vi "FGV_RichText.vi"(11 ".NET Refnum in":refnum<k24>) -> ()   [LabVIEW 2017]
uses:
  System.Windows.Forms
panel:
  out "error out":errorcluster
  in  "error in (no error)":errorcluster
  in  "FV":T1(ring)
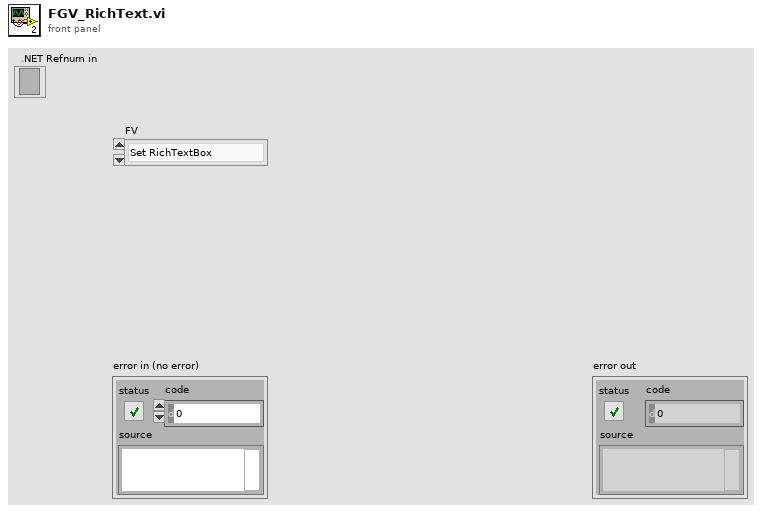
[diagram p1: front panel]
types:
  T1 = enum16{"Set RichTextBox", "LoadRTFFile", "Undo", "Redo", "Copy", "Cut", "Past", "Clear", "Find", "Save", "Initialize"}
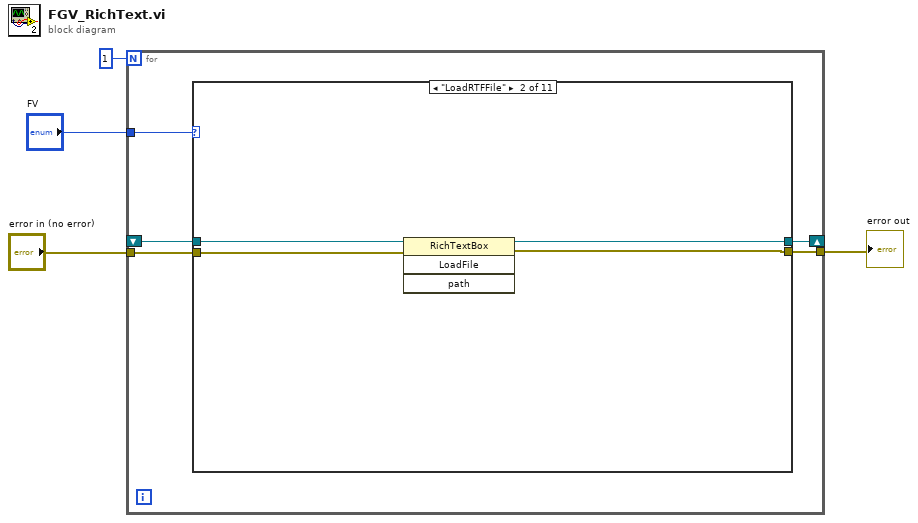
[diagram p0: block diagram]
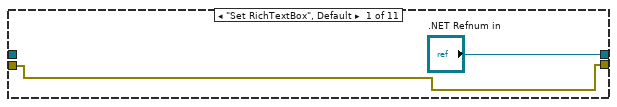
[diagram p2: hidden frame]
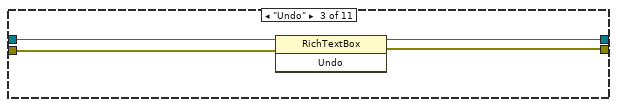
[diagram p3: hidden frame]
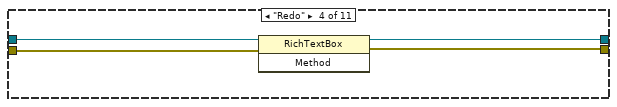
[diagram p4: hidden frame]
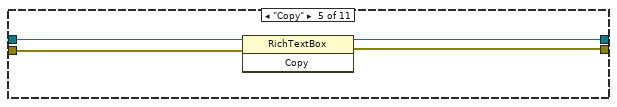
[diagram p5: hidden frame]
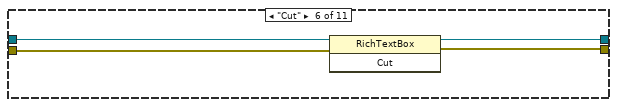
[diagram p6: hidden frame]
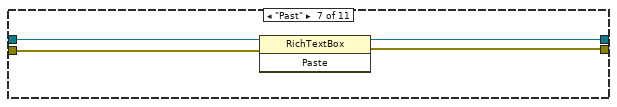
[diagram p7: hidden frame]
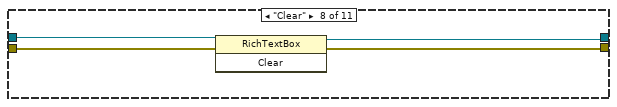
[diagram p8: hidden frame]
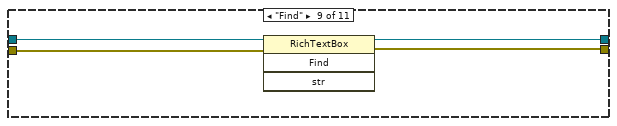
[diagram p9: hidden frame]
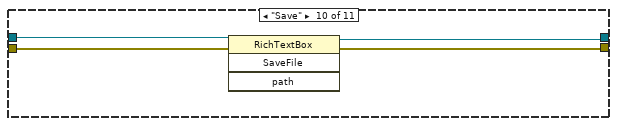
[diagram p10: hidden frame]
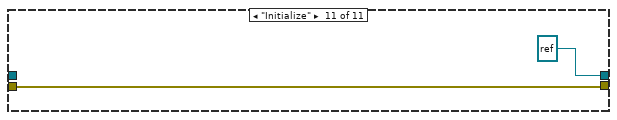
[diagram p11: hidden frame]
diagram:
  n1 = for {
    N: 1 -> [_]
    tunnel: "FV" -> [w9]
    shift-right: [w8] -> _
    shift-left: _ -> [w7]
    tunnel: [w6] -> w2
    tunnel: "error in (no error)" -> [w5]
    n2 = case shown="\"LoadRTFFile\"" w9 {
      tunnel: [".NET Refnum in" w12 w18 w21 w25 w29 w33 w37 w41 w45 refnum<k24> refnum (".NET Refnum in")] -> w8
      tunnel: w7 -> [_ w15 w19 w23 w27 w31 w35 w39 w43 w47 _]
      tunnel: [w10 w14 w17 w20 w24 w28 w32 w36 w40 w44 w49] -> w6
      tunnel: w5 -> [w10 w13 w16 w22 w26 w30 w34 w38 w42 w46 w49]
      frame "Set RichTextBox", Default {
      }
      frame "LoadRTFFile" {
        n3 = invoke class="RichTextBox" method="LoadFile"(reference=w15, error in=w13) -> (reference out=w12:refnum<k24>, error out=w14:errorcluster)  [unwired: 2 in, 2 out]
      }
      frame "Undo" {
        n4 = invoke class="RichTextBox" method="Undo"(reference=w19, error in=w16) -> (reference out=w18:refnum<k24>, error out=w17:errorcluster)  [unwired: 1 in, 1 out]
      }
      frame "Redo" {
        n5 = invoke class="RichTextBox" method=#-1(reference=w23, error in=w22) -> (reference out=w21:refnum<k24>, error out=w20:errorcluster)  [unwired: 1 in, 1 out]
      }
      frame "Copy" {
        n6 = invoke class="RichTextBox" method="Copy"(reference=w27, error in=w26) -> (reference out=w25:refnum<k24>, error out=w24:errorcluster)  [unwired: 1 in, 1 out]
      }
      frame "Cut" {
        n7 = invoke class="RichTextBox" method="Cut"(reference=w31, error in=w30) -> (reference out=w29:refnum<k24>, error out=w28:errorcluster)  [unwired: 1 in, 1 out]
      }
      frame "Past" {
        n8 = invoke class="RichTextBox" method="Paste"(reference=w35, error in=w34) -> (reference out=w33:refnum<k24>, error out=w32:errorcluster)  [unwired: 1 in, 1 out]
      }
      frame "Clear" {
        n9 = invoke class="RichTextBox" method="Clear"(reference=w39, error in=w38) -> (reference out=w37:refnum<k24>, error out=w36:errorcluster)  [unwired: 1 in, 1 out]
      }
      frame "Find" {
        n10 = invoke class="RichTextBox" method="Find"(reference=w43, error in=w42) -> (reference out=w41:refnum<k24>, error out=w40:errorcluster)  [unwired: 2 in, 2 out]
      }
      frame "Save" {
        n11 = invoke class="RichTextBox" method="SaveFile"(reference=w47, error in=w46) -> (reference out=w45:refnum<k24>, error out=w44:errorcluster)  [unwired: 2 in, 2 out]
      }
      frame "Initialize" {
      }
    }
  }
  "error out" <- w2
